vi "Balance Loop.vi"(8 "error in (no error)":errorcluster, 9 "PID gains":T1={"proportional gain (Kc)"=-4.8049, "integral time (Ti, min)"=50.38629, "derivative time (Td, min)"=0.000943} {"derivative time (Td, min)" format="%.3f"; "integral time (Ti, min)" format="%.3f"; "proportional gain (Kc)" format="%.3f"}, 10 "maxDiff":dbl=0.75, 11 "Refnum in":refnum<k20>) -> (0 "error out":errorcluster, 3 "Refnum Out":refnum<k20>)   [LabVIEW 2016]
uses:
  <vilib>/Platform/TimedLoop/XDataNode/timing_clust.ctl
  <vilib>/Platform/TimedLoop/XDataNode/nitl_modes.ctl
  <vilib>/Platform/TimedLoop/XDataNode/wakeup.ctl
  Typedef/Remote Control Cluster.ctl
  Typedef/INS Data.ctl
  Shared resoruces/Navigation Variables.vi
  Shared resoruces/Front Panel Control Variables.vi
  <vilib>/addons/control/pid/pid.llb/PID (DBL).vi
  <vilib>/Utility/error.llb/Error Cluster From Error Code.vi
  <vilib>/rvi/errors/niLvFpgaAdjustHostInterfaceError.vi
  <vilib>/RVI Host/nirviSupport.llb/nirviErrorClusterFromErrorCode.vi
  <vilib>/platform/TimedLoop/XDataNode/XDataNode.xnode
  <vilib>/rvi/interface/nirviMethod/nirviMethod.xnode
  <vilib>/rvi/interface/nirviReadWriteControl/nirviReadWriteControl.xnode
  NiFpgaLv.dll
  <vilib>/rvi/interface/Simulation/niFpgaSimulationCallBeginRW.vi
  <vilib>/FPGAPlugInAG/Dynamic/niLvFpga_WriteFifo_Dynamic.vi
  <vilib>/rvi/errors/niLvFpgaMergeErrorWithErrorCode.vi
  <vilib>/rvi/interface/nirviMethod/StockFPGA_InlinedMethodWaitForSingleIRQ.vi
  <vilib>/FPGAPlugInAG/Dynamic/niLvFpga_WaitOnIrq_Dynamic.vi
  <vilib>/FPGAPlugInAG/Dynamic/niLvFpga_AcknowledgeIrq_Dynamic.vi
  <vilib>/addons/control/pid/NI_PID_pid.lvlib
  Shared resoruces/Shared resources RT.lvlib
  <vilib>/Platform/TimedLoop/XDataNode/XDNodeRunTimeDep.lvlib
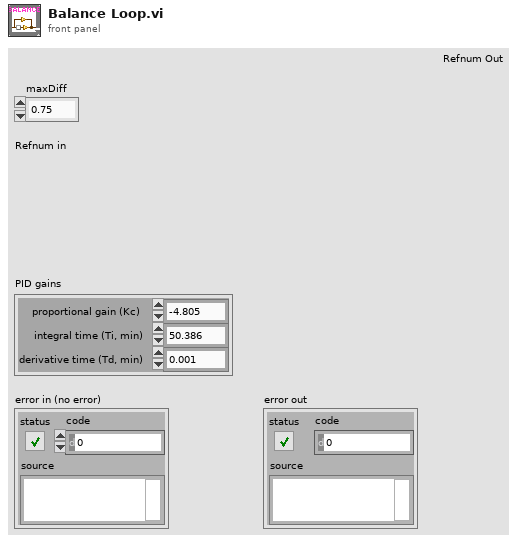
[diagram p1: front panel]
types:
  T1 = cluster{"proportional gain (Kc)":dbl, "integral time (Ti, min)":dbl, "derivative time (Td, min)":dbl}
  T2 = typedef "XDNodeRunTimeDep.lvlib/timing_clust.ctl" = cluster{"Expected End [f-1]":u64, "Actual End [f-1]":u64, "Finished Late? [f-1]":bool, "Expected End [i-1]":u64, "Actual End [i-1]":u64, "Finished Late? [i-1]":bool, "Expected Start [i]":u64, "Actual Start [i]":u64, "Expected Start [f]":u64, "Actual Start [f]":u64, "Source Name":string, "Structure Name":string, "Period":i64, "Deadline":i64, "Offset":i64, "Start":i64, "Priority":i32, "Timeout":i32, "Mode":T3, "Wakeup Reason":T4, "Error":errorcluster, "Source Type":string, "Secondary Source Type":string, "Global End Time":u64, "Global Start Time":u64, "Frame Duration":u64, "Iteration Duration":u64, "Assigned CPU":i32, "I/O Scan Engine Mode":u32}
  T3 = typedef "XDNodeRunTimeDep.lvlib/nitl_modes.ctl" = enum32{"No Change", "Process missed periods, maintain original phase", "Discard missed periods, maintain original phase", "Process missed periods, ignore original phase", "Discard missed periods, ignore original phase"}
  T4 = typedef "XDNodeRunTimeDep.lvlib/wakeup.ctl" = enum32{"Normal", "Aborted", "Asynchronous wakeup", "Timing source error", "Timed loop error", "Timeout"}
  T5 = typedef "Remote Control Cluster.ctl" = cluster{"Pot1":u16, "Pot2":u16, "Pot3":u16, "Pot4":u16, "Switch1":cluster{"L":bool, "H":bool}, "Switch2":cluster{"L":bool, "H":bool}, "Switch3":cluster{"L":bool, "H":bool}}
  T6 = typedef "INS Data.ctl" = cluster{"Yaw":sgl, "Pitch":sgl, "Roll":sgl, "Lat":dbl, "Long":dbl, "Alt":dbl, "North":dbl, "East":dbl, "Down":dbl, "PosU":dbl, "VelU":dbl}
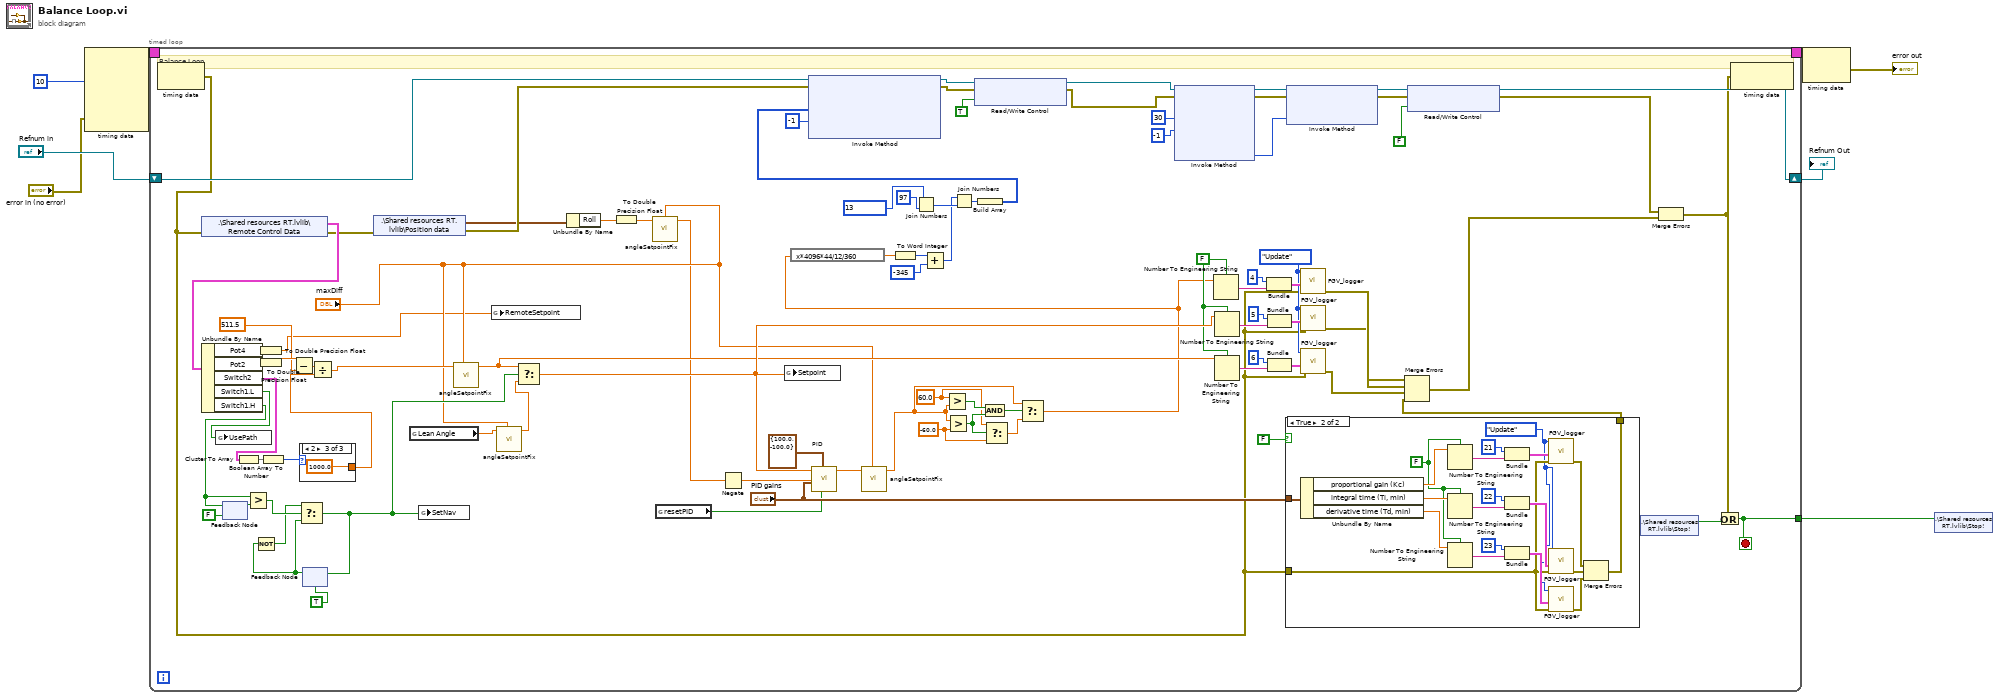
[diagram p0: block diagram]
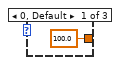
[diagram p3: hidden frame]
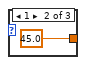
[diagram p4: hidden frame]
diagram:
  n1 = node-c288(i64 10 ("Period"), "error in (no error)") -> (w5:T2)  [unwired: 3 in]
  n2 = timed-loop {
    shift-right: [w99] -> w6
    shift-left: "Refnum in" -> [w100]
    tunnel: [w68] -> w7
    timing: w5 -> [_]
    timing-out: [_] -> w4
    stop <- w68 stop-if-true
    w16 = -60.0
    w17 = 60.0
    w27 = enum16{"Update", "Log", "Init"}."Update" ("Command")
    w33 = FALSE ("use system decimal point (T)")
    # "Balance Loop"
    n3 = node-c288() -> (w24:errorcluster)  [unwired: 1 in]
    n4 = shared-variable ".\\Shared resources RT.lvlib\\Remote Control Data"(error in=w24) -> (w67:T5, error out=w62:errorcluster)
    n5 = Unbundle By Name(w67) -> ("Pot4"=w22:u16, "Pot2"=w98:u16, "Switch2"=w66:cluster{"L":bool, "H":bool}, "Switch1.L"=w25:bool, "Switch1.H"=w26:bool)
    n6 = global write "Navigation Variables.vi" "UsePath"(w25) -> ()
    n7 = feedback-in #1(w26) -> ()
    n8 = feedback #1(FALSE ("H")) -> (w48:bool)
    n9 = Cluster To Array(cluster=w66) -> (array=w65:bool[])
    n10 = Greater?(x=w26, y=w48) -> (0:w46:bool)
    n11 = To Double Precision Float(number=w22) -> (double precision float=w9:dbl)
    n12 = To Double Precision Float(number=w98) -> (double precision float=w96:dbl)
    n13 = Boolean Array To Number(Boolean array=w65) -> (number=w64:u32)
    n14 = Subtract(x=w96, y=511.5 ("x")) -> (x-y=w97:dbl)
    n15 = case shown="2" w64 {
      tunnel: [100.0 45.0 1000.0] -> w63
      frame 0, Default {
      }
      frame 1 {
      }
      frame 2 {
      }
    }
    n16 = feedback #2(TRUE) -> (w44:bool)
    n17 = Not(x=w44) -> (.not. x?=w43:bool)
    n18 = Select(t=w43, s=w46, f=w44) -> (s? t:f=w37:bool)
    n19 = feedback-in #2(w37) -> ()
    n20 = Divide(x=w97, y=w63) -> (x/y=w29:dbl)
    n21 = shared-variable ".\\Shared resources RT.lvlib\\Position data"(error in=w62) -> (w60:T6, error out=w61:errorcluster)
    n22 = global read "Navigation Variables.vi" "Lean Angle"() -> (w39:dbl)
    n23 = global write "Navigation Variables.vi" "SetNav"(w37) -> ()
    n24 = call "angleSetpointFix.vi"("maxDiff"="maxDiff", "Angle in"=w29) -> ("Angle out"=w28:dbl)  [unwired: 9 in]
    n25 = global write "Navigation Variables.vi" "RemoteSetpoint"(w9) -> ()
    n26 = call "angleSetpointFix.vi"("maxDiff"="maxDiff", "Angle in"=w39) -> ("Angle out"=w38:dbl)  [unwired: 9 in]
    n27 = Select(t=w28, s=w37, f=w38) -> (s? t:f=w41:dbl)
    n28 = Unbundle By Name(w60) -> ("Roll"=w13:sgl)
    n29 = To Double Precision Float(number=w13) -> (double precision float=w10:dbl)
    n30 = call "angleSetpointFix.vi"("maxDiff"="maxDiff", "Angle in"=w10) -> ("Angle out"=w11:dbl)  [unwired: 9 in]
    n31 = global read "Front Panel Control Variables.vi" "resetPID"() -> (w40:bool)
    n32 = Negate(x=w11) -> (-x=w71:dbl)
    n33 = global write "Navigation Variables.vi" "Setpoint"(w41) -> ()
    n34 = call-poly <vilib>:"PID.vi"("reinitialize? (F)"=w40, "output range"=cluster{"output high":dbl, "output low":dbl} {"output high"=100.0, "output low"=-100.0}, "PID gains"="PID gains", "process variable"=w71, "setpoint"=w41) -> ("output"=w70:dbl)  [unwired: 5 in, 1 out]
    n35 = call "angleSetpointFix.vi"("maxDiff"="maxDiff", "Angle in"=w70) -> ("Angle out"=w19:dbl)  [unwired: 9 in]
    n36 = Join Numbers(hi=u8 13 ("lo"), lo=u8 97) -> ((hi.lo)=w79:u16)
    n37 = Greater?(x=w17, y=w19) -> (0:w21:bool)
    n38 = Greater?(x=w19, y=w16) -> (0:w18:bool)
    n39 = And(x=w21, y=w18) -> (x .and. y?=w20:bool)
    n40 = Select(t=w17, s=w18, f=w16) -> (s? t:f=w15:dbl)
    n41 = Select(t=w19, s=w20, f=w15) -> (s? t:f=w14:dbl)
    n42 = expression code="x*4096*44/12/360"(w14) -> (w73:dbl)
    n43 = To Word Integer(number=w73) -> (16bit integer=w76:i16)
    n44 = Add(x=w76, y=i16 -345 ("hi")) -> (x+y=w74:i16)
    n45 = Join Numbers(hi=w74, lo=w79) -> ((hi.lo)=w78:u32)
    n46 = Build Array(w78) -> (w75:u32[])
    n47 = xnode "Invoke Method"("FPGA VI Reference In"=w100, "error in"=w61, "Data"=w75, "Timeout (ms)"=-1) -> ("FPGA VI Reference Out"=w87:refnum<k20>, "error out"=w88:errorcluster)  [unwired: 1 out]
    n48 = xnode "Read/Write Control"("FPGA VI Reference In"=w87, "error in"=w88, "ODrive RT Control"=TRUE) -> ("FPGA VI Reference Out"=w86:refnum<k20>, "error out"=w85:errorcluster)
    n49 = xnode "Invoke Method"("FPGA VI Reference In"=w86, "error in"=w85, "IRQ Number(s)"=30, "Timeout (ms)"=-1) -> ("FPGA VI Reference Out"=w94:refnum<k20>, "error out"=w93:errorcluster, "IRQ(s) Asserted"=w83:i32)  [unwired: 1 out]
    n50 = Number To Engineering String(1:w33, 4:w14) -> (0:w57:string)  [unwired: 2 in]
    n51 = Number To Engineering String(1:w33, 4:w41) -> (0:w54:string)  [unwired: 2 in]
    n52 = Number To Engineering String(1:w33, 4:w28) -> (0:w34:string)  [unwired: 2 in]
    n53 = Bundle(4, w57) -> (w58:cluster{i32, string})  [unwired: 1 in]
    n54 = Bundle(5, w54) -> (w55:cluster{i32, string})  [unwired: 1 in]
    n55 = Bundle(6, w34) -> (w35:cluster{i32, string})  [unwired: 1 in]
    n56 = case shown="True" FALSE {
      tunnel: "PID gains" -> [_ w123]
      tunnel: w24 -> [w106 w112]
      tunnel: [w106 w108] -> w31
      frame False {
      }
      frame True {
        w107 = enum16{"Update", "Log", "Init"}."Update" ("Command")
        w113 = FALSE ("use system decimal point (T)")
        n57 = Unbundle By Name(w123) -> ("proportional gain (Kc)"=w122:dbl, "integral time (Ti, min)"=w115:dbl, "derivative time (Td, min)"=w114:dbl)
        n58 = Number To Engineering String(1:w113, 4:w122) -> (0:w124:string)  [unwired: 2 in]
        n59 = Number To Engineering String(1:w113, 4:w115) -> (0:w119:string)  [unwired: 2 in]
        n60 = Number To Engineering String(1:w113, 4:w114) -> (0:w116:string)  [unwired: 2 in]
        n61 = Bundle(21, w124) -> (w125:cluster{i32, string})  [unwired: 1 in]
        n62 = Bundle(22, w119) -> (w120:cluster{i32, string})  [unwired: 1 in]
        n63 = Bundle(23, w116) -> (w117:cluster{i32, string})  [unwired: 1 in]
        n64 = call "FGV_logger.vi"("error in"=w112, 9:w125, "Command"=w107) -> ("error out"=w111:errorcluster)  [unwired: 8 in]
        n65 = call "FGV_logger.vi"("error in"=w112, 9:w120, "Command"=w107) -> ("error out"=w110:errorcluster)  [unwired: 8 in]
        n66 = call "FGV_logger.vi"("error in"=w112, 9:w117, "Command"=w107) -> ("error out"=w109:errorcluster)  [unwired: 8 in]
        n67 = Merge Errors(w111, w110, w109) -> (w108:errorcluster)
      }
    }
    n68 = xnode "Invoke Method"("FPGA VI Reference In"=w94, "error in"=w93, "IRQ Number(s)"=w83) -> ("FPGA VI Reference Out"=w91:refnum<k20>, "error out"=w82:errorcluster)
    n69 = call "FGV_logger.vi"("error in"=w24, 9:w58, "Command"=w27) -> ("error out"=w53:errorcluster)  [unwired: 8 in]
    n70 = call "FGV_logger.vi"("error in"=w24, 9:w55, "Command"=w27) -> ("error out"=w52:errorcluster)  [unwired: 8 in]
    n71 = call "FGV_logger.vi"("error in"=w24, 9:w35, "Command"=w27) -> ("error out"=w30:errorcluster)  [unwired: 8 in]
    n72 = Merge Errors(w53, w52, w30, w31) -> (w50:errorcluster)
    n73 = xnode "Read/Write Control"("FPGA VI Reference In"=w91, "error in"=w82, "ODrive RT Control"=FALSE) -> ("FPGA VI Reference Out"=w99:refnum<k20>, "error out"=w51:errorcluster)
    n74 = shared-variable ".\\Shared resources RT.lvlib\\Stop!"() -> (w69:bool)  [unwired: 1 in, 1 out]
    n75 = Merge Errors(w51, w50) -> (w23:errorcluster)
    n76 = Or(x=w23, y=w69) -> (x .or. y?=w68:bool)
    n77 = node-c288(w23) -> ()  [unwired: 1 out]
  }
  "Refnum Out" <- w6
  n78 = node-c288(w4) -> (→"error out":errorcluster)
  n79 = shared-variable ".\\Shared resources RT.lvlib\\Stop!"(w7) -> ()  [unwired: 1 in, 1 out]
